vi "IFNoise-Update AO.vi"(0 "Runtime":T1, 11 "error in (no error)":errorcluster) -> (15 "error out":errorcluster)   [LabVIEW 2015]
uses:
  Type Defs/IFNoise-Runtime.ctl
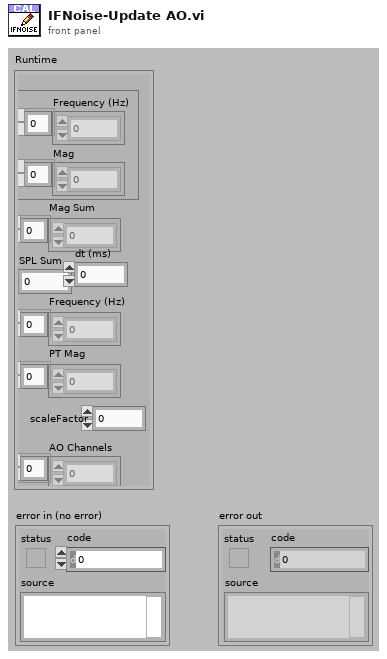
[diagram p1: front panel]
types:
  T1 = typedef "IFNoise-Runtime.ctl" = cluster{"Calibration":cluster{"Frequency (Hz)":dbl[], "Mag":dbl[]}, "Mag Sum":dbl[], "SPL Sum":dbl, "Frequency (Hz)":dbl[], "PT Mag":dbl[], "dt (ms)":dbl, "AO Channels":i32[], "scaleFactor":dbl}
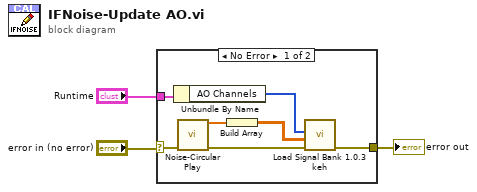
[diagram p0: block diagram]
diagram:
  n1 = case shown="No Error" "error in (no error)" {
    selector: "error in (no error)" -> [w9 w11]
    tunnel: [w4 w11] -> w2
    tunnel: "Runtime" -> [w10 _]
    frame No Error {
      n2 = Unbundle By Name(w10) -> ("AO Channels"=w5:i32[])
      n3 = call "Noise-Circular Play.vi"("error in (no error)"=w9) -> ("Noise (out)"=w7:dbl[], "error out"=w8:errorcluster)  [unwired: 13 in]
      n4 = Build Array(w7) -> (w6:dbl[][])
      n5 = call "Load Signal Bank 1.0.3 keh.vi"("error in (no error)"=w8, "Input array"=w6, "Active AO Array"=w5) -> ("error out"=w4:errorcluster)  [unwired: 3 in, 1 out]
    }
    frame Error {
    }
  }
  "error out" <- w2
